vi "set Tables Flag from SPANIdx.vi"(11 "SPAN Idx":i32) -> (3 "set Tables":bool)   [LabVIEW 2020, in "Linearisierung v2.lvlib" / "SpanEinstellungen.lvlib"]
uses:
  SpanEinstellungen.lvlib
  Aktion FGV Spans abarbeiten.ctl
  Aktion FGV SpanEinstellungen.ctl
  Gasteiler/Aktionen FGV Gasteiler Daten.ctl
  Gasteiler/Gasteiler.lvlib
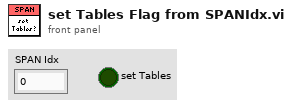
[diagram p1: front panel]
types:
  T1 = typedef "Linearisierung v2.lvlib/Gasteiler.lvlib/Aktionen FGV Gasteiler Daten.ctl" = enum16{"lesen", "Gasteiler Daten", "Seriellen Param.", "MB-Endwert", "laden", "speichern", "Anforderung", "TCP", "Aufzeichnung Start"}
  T2 = typedef "Linearisierung v2.lvlib/SpanEinstellungen.lvlib/Aktion FGV SpanEinstellungen.ctl" = enum16{"lesen", "schreiben", "laden", "speichern", "RegisterRef", "automatisch", "init", "PDF Params", "Punkte umkehren"}
  T3 = typedef "Linearisierung v2.lvlib/SpanEinstellungen.lvlib/Aktion FGV Spans abarbeiten.ctl" = enum16{"lesen", "idle", "start", "next", "comp", "init", "running", "abort"}
  T4 = typedef "System Einstellungen V2.lvlib/Konfig Gasflasche.ctl" = bool
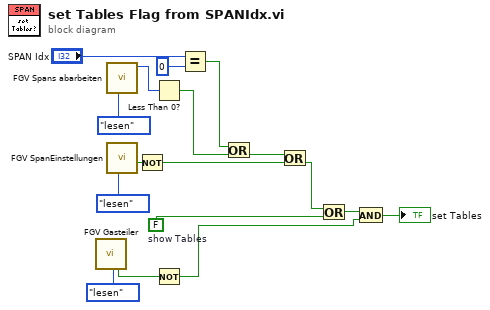
[diagram p0: block diagram]
diagram:
  w17 = FALSE  # show Tables
  n1 = call "FGV Gasteiler.vi"("Aktionen"=Aktionen_FGV_Gasteiler_Daten."lesen") -> ("Aufzeichnung Start"=w3:bool)  [unwired: 11 in, 7 out]
  n2 = call "FGV Spans abarbeiten.vi"("Aktion"=Aktion_FGV_Spans_abarbeiten."lesen") -> ("active SPAN Idx out"=w8:i32)  [unwired: 5 in, 5 out]
  n3 = call "FGV SpanEinstellungen.vi"("Aktion"=Aktion_FGV_SpanEinstellungen."lesen") -> ("automatisch out"=w13:T4)  [unwired: 6 in, 4 out]
  n4 = Not(x=w13) -> (.not. x?=w12:T4)
  n5 = Less Than 0?(x=w8) -> (x < 0?=w7:bool)
  n6 = Not(x=w3) -> (.not. x?=w6:bool)
  n7 = Equal?(x="SPAN Idx", y=0) -> (x = y?=w10:bool)
  n8 = Or(x=w10, y=w7) -> (x .or. y?=w9:bool)
  n9 = Or(x=w9, y=w12) -> (x .or. y?=w11:T4)
  n10 = Or(x=w11, y=w17) -> (x .or. y?=w14:T4)
  n11 = And(x=w14, y=w6) -> (x .and. y?=→"set Tables":T4)
